vi "VIPM Repositories--constant.vi"() -> (2 "Index Filenames":string[](array[string]), 3 "Repo URLs":string[](array[string]))   [LabVIEW 2016, in "Packages.lvlib" / "VIPM.lvlib"]
uses:
  VIPM.lvlib
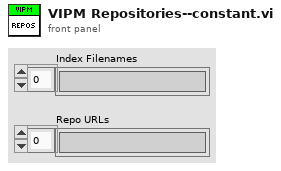
[diagram p1: front panel]
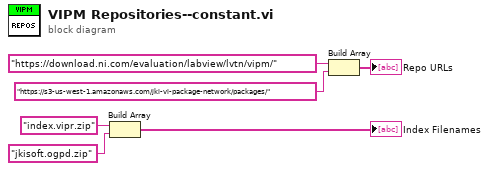
[diagram p0: block diagram]
diagram:
  n1 = Build Array("index.vipr.zip" ("Repo URL"), "jkisoft.ogpd.zip" ("Repo URL")) -> (→"Index Filenames":string[])
  n2 = Build Array("https://download.ni.com/evaluation/labview/lvtn/vipm/" ("Repo URL"), "https://s3-us-west-1.amazonaws.com/jki-vi-package-network/packages/" ("Repo URL")) -> (→"Repo URLs":string[])
